vi "getParam_array.vi"(8 "error in (no error)":errorcluster, 11 "ScriptEvent in":refnum<class "ScriptEvent.lvclass">) -> (0 "error out":errorcluster, 2 "param_array":T1(array[cluster]), 3 "ScriptEvent out":refnum<class "ScriptEvent.lvclass">)   [LabVIEW 2011, in "Tools.lvlib" / "Scripting.lvlib" / "ScriptEvent.lvclass"]
uses:
  ScriptEvent.lvclass
  ScriptEvent.lvclass/ScriptEvent.ctl
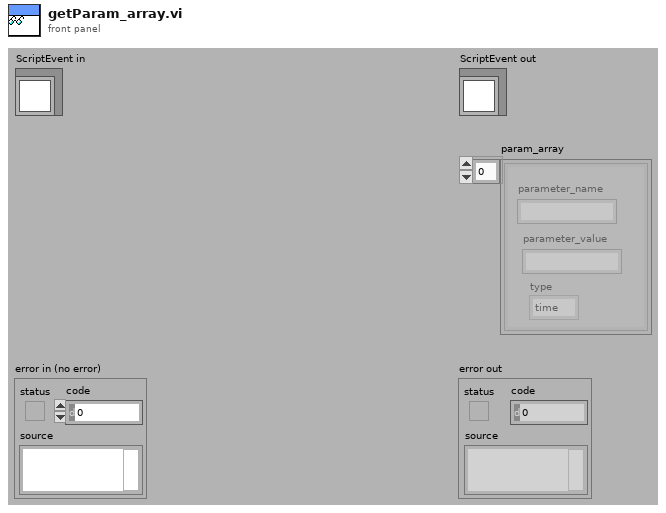
[diagram p1: front panel]
types:
  T1 = cluster{"parameter_name":string, "parameter_value":string, "type":enum16{"time", "time_difference", "value", "frequency", "phase", "ramp_time", "value_step", "time_step", "number_of_steps", "start_value", "end_value", "start_freq", "start_amp", "start_phase", "end_freq", "end_amp", "end_phase"}}[]
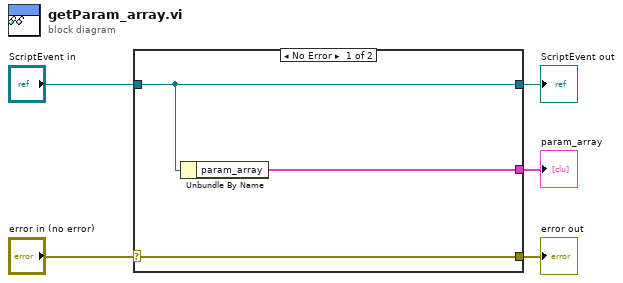
[diagram p0: block diagram]
diagram:
  n1 = case shown="No Error" "error in (no error)" {
    selector: "error in (no error)" -> [w8 w9]
    tunnel: [w8 w9] -> w4
    tunnel: [w7 w10] -> w2
    tunnel: "ScriptEvent in" -> [w7 w10]
    tunnel: [w6 _] -> w1
    frame No Error {
      n2 = Unbundle By Name(w7) -> ("param_array"=w6:T1)
    }
    frame Error {
    }
  }
  "error out" <- w4
  "ScriptEvent out" <- w2
  "param_array" <- w1
